vi "LaudaLedCtrl2.vi"(9 "ctrl_mode":dbl, 10 "T ext / T ext in":enum32{"Sensor 1", "Sensor 2"}(radio)) -> (1 "Sensor OK 5":bool, 2 "Sensor OK 3":bool, 3 "Sensor OK 4":bool, 4 "Sensor OK 6":bool)   [LabVIEW 2016]
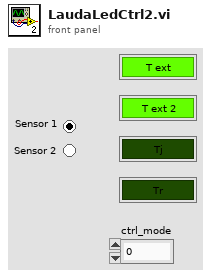
[diagram p1: front panel]
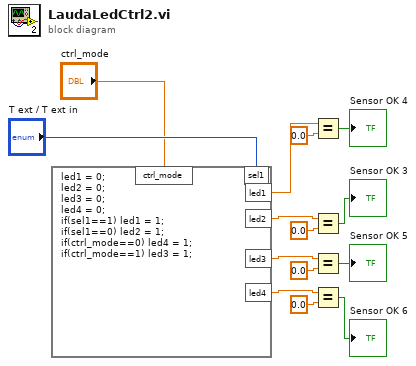
[diagram p0: block diagram]
diagram:
  n1 = formula code="led1 = 0;\nled2 = 0;\nled3 = 0;\nled4 = 0;\nif(sel1==1) led1 = 1;\nif(sel1==0) led2 = 1;\nif(ctrl_mode==0) led4 = 1;\nif(ctrl_mode==1) led3 = 1;"("sel1"="T ext / T ext in", "ctrl_mode"="ctrl_mode") -> ("led1"=w3:dbl, "led2"=w5:dbl, "led3"=w10:dbl, "led4"=w11:dbl)
  n2 = Equal?(x=w3, y=0.0) -> (x = y?=→"Sensor OK 4":bool)
  n3 = Equal?(x=w5, y=0.0) -> (x = y?=→"Sensor OK 3":bool)
  n4 = Equal?(x=w10, y=0.0) -> (x = y?=→"Sensor OK 5":bool)
  n5 = Equal?(x=w11, y=0.0) -> (x = y?=→"Sensor OK 6":bool)
